vi "Unregister Actor.vi"(8 "error in (no error)":errorcluster, 10 "Index":i32=-1, 11 "cRIO-CO2 in":refnum<class "cRIO-CO2.lvclass">) -> (0 "error out":errorcluster, 3 "cRIO-CO2 out":refnum<class "cRIO-CO2.lvclass">)   [LabVIEW 2015, in "cRIO-Carbondioxide.lvlib" / "cRIO-CO2.lvlib" / "cRIO-CO2.lvclass"]
uses:
  cRIO-CO2.lvclass
  cRIO-CO2.lvclass/cRIO-CO2.ctl
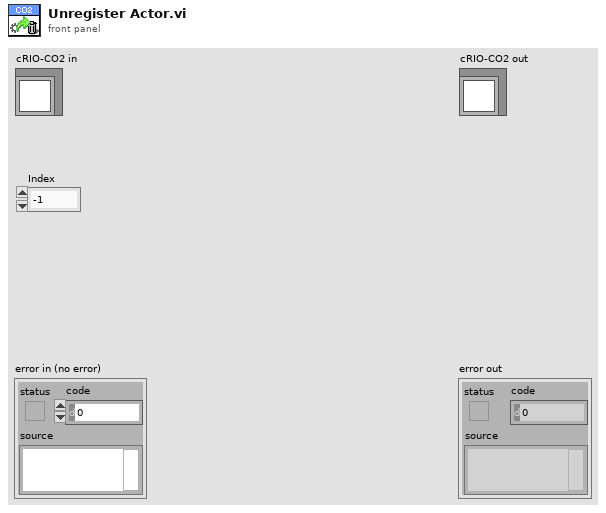
[diagram p1: front panel]
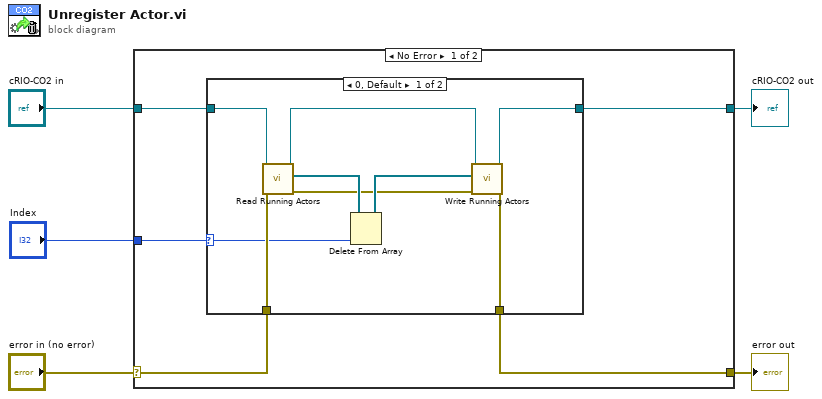
[diagram p0: block diagram]
diagram:
  n1 = case shown="No Error" "error in (no error)" {
    selector: "error in (no error)" -> [w7 w23]
    tunnel: [w9 w23] -> w4
    tunnel: [w8 w22] -> w2
    tunnel: "cRIO-CO2 in" -> [w10 w22]
    tunnel: "Index" -> [w6 _]
    frame No Error {
      n2 = case shown="0, Default" w6 {
        selector: w6 -> [w12 _]
        tunnel: w10 -> [w18 w21]
        tunnel: [w17 w20] -> w9
        tunnel: [w14 w21] -> w8
        tunnel: w7 -> [w13 w20]
        frame 0, Default {
          n3 = call "Read Running Actors.vi"("error in (no error)"=w13, "cRIO-CO2 in"=w18) -> ("error out"=w11:errorcluster, "Running Actors"=w19:refnum<class "CO2 Actor.lvclass">[], "cRIO-CO2 out"=w15:refnum<class "cRIO-CO2.lvclass">)  [unwired: 7 in]
          n4 = Delete From Array(array=w19, index=w12) -> (array with subset deleted=w16:refnum<class "CO2 Actor.lvclass">[])  [unwired: 1 in, 1 out]
          n5 = call "Write Running Actors.vi"("error in (no error)"=w11, "Running Actors"=w16, "cRIO-CO2 in"=w15) -> ("error out"=w17:errorcluster, "cRIO-CO2 out"=w14:refnum<class "cRIO-CO2.lvclass">)  [unwired: 7 in]
        }
        frame -1 {
        }
      }
    }
    frame Error {
    }
  }
  "error out" <- w4
  "cRIO-CO2 out" <- w2
